vi "Outputs.vi"() -> ()   [LabVIEW 2017]
panel:
  in  "alpha":i16 max=1023
  in  "J":i16 max=1023
  in  "Grip":i16 max=1023
  in  "Z":i16 max=1023
  in  "R":i16 max=1023
  in  "teta":i16 max=1023
  in  "dy_counter":i8
  in  "LED":i8
  in  "Vp":dbl
  in  "Vy":dbl
  in  "Vx":dbl
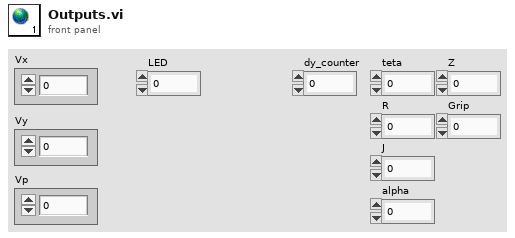
[diagram p1: front panel]
diagram:
